vi "5 ch 12kHz only esonance scanner (FPGA) fixed pix clock.vi"() -> ()   [LabVIEW 2012]
uses:
  <vilib>/Platform/TimedLoop/XDataNode/timing_clust.ctl
  <vilib>/Platform/TimedLoop/XDataNode/nitl_modes.ctl
  <vilib>/Platform/TimedLoop/XDataNode/wakeup.ctl
  <vilib>/rvi/eio/common/nirviEmuTemplateMethod_errors.vi
  <vilib>/rvi/Emulation/niFpgaSctlEmulationRegisterWithScheduler.vi
  <vilib>/rvi/interface/RandomDataEmulation/nirviRandomDataFPGAFIFO.vi
  <vilib>/rvi/interface/RandomDataEmulation/niFpgaRandomDataHandleErrors.vi
  <vilib>/rvi/Emulation/niFpgaSctlEmulationScheduler.vi
  <vilib>/eio/EIONode/EIONode.xnode
  <vilib>/Platform/TimedLoop/XDataNode/XDataNode.xnode
  <vilib>/rvi/DataTransferAndStorage/Container/XNode/niFpgaContainer.xnode
  <vilib>/rvi/interface/RandomDataEmulation/nirviRandomDataFpgaReadWriteTemplate.vi
  <vilib>/Platform/TimedLoop/XDataNode/XDNodeRunTimeDep.lvlib
panel:
  in  "frequency (T:8kHz F:12kHz)":bool
  in  "lines at once":i16=4999
  in  "Start Delay (Ticks)":i16 caption="Start delay (Ticks)"
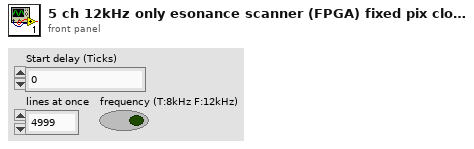
[diagram p1: front panel]
types:
  T1 = typedef "XDNodeRunTimeDep.lvlib/timing_clust.ctl" = cluster{"Expected End [f-1]":u64, "Actual End [f-1]":u64, "Finished Late? [f-1]":bool, "Expected End [i-1]":u64, "Actual End [i-1]":u64, "Finished Late? [i-1]":bool, "Expected Start [i]":u64, "Actual Start [i]":u64, "Expected Start [f]":u64, "Actual Start [f]":u64, "Source Name":string, "Structure Name":string, "Period":i64, "Deadline":i64, "Offset":i64, "Start":i64, "Priority":i32, "Timeout":i32, "Mode":T2, "Wakeup Reason":T3, "Error":errorcluster, "Source Type":string, "Secondary Source Type":string, "Global End Time":u64, "Global Start Time":u64, "Frame Duration":u64, "Iteration Duration":u64, "Assigned CPU":i32, "I/O Scan Engine Mode":u32}
  T2 = typedef "XDNodeRunTimeDep.lvlib/nitl_modes.ctl" = enum32{"No Change", "Process missed periods, maintain original phase", "Discard missed periods, maintain original phase", "Process missed periods, ignore original phase", "Discard missed periods, ignore original phase"}
  T3 = typedef "XDNodeRunTimeDep.lvlib/wakeup.ctl" = enum32{"Normal", "Aborted", "Asynchronous wakeup", "Timing source error", "Timed loop error", "Timeout"}
  T4 = cluster{"IO Module\\AI A0":i16, "IO Module\\AI A1":i16, "IO Module\\AI A3":i16, "IO Module\\AI A6":i16, "IO Module\\AI B8":i16}
  T5 = cluster{"IO Module\\AI A0":i32, "IO Module\\AI A1":i32, "IO Module\\AI A3":i32, "IO Module\\AI A6":i32, "IO Module\\AI B8":i32}
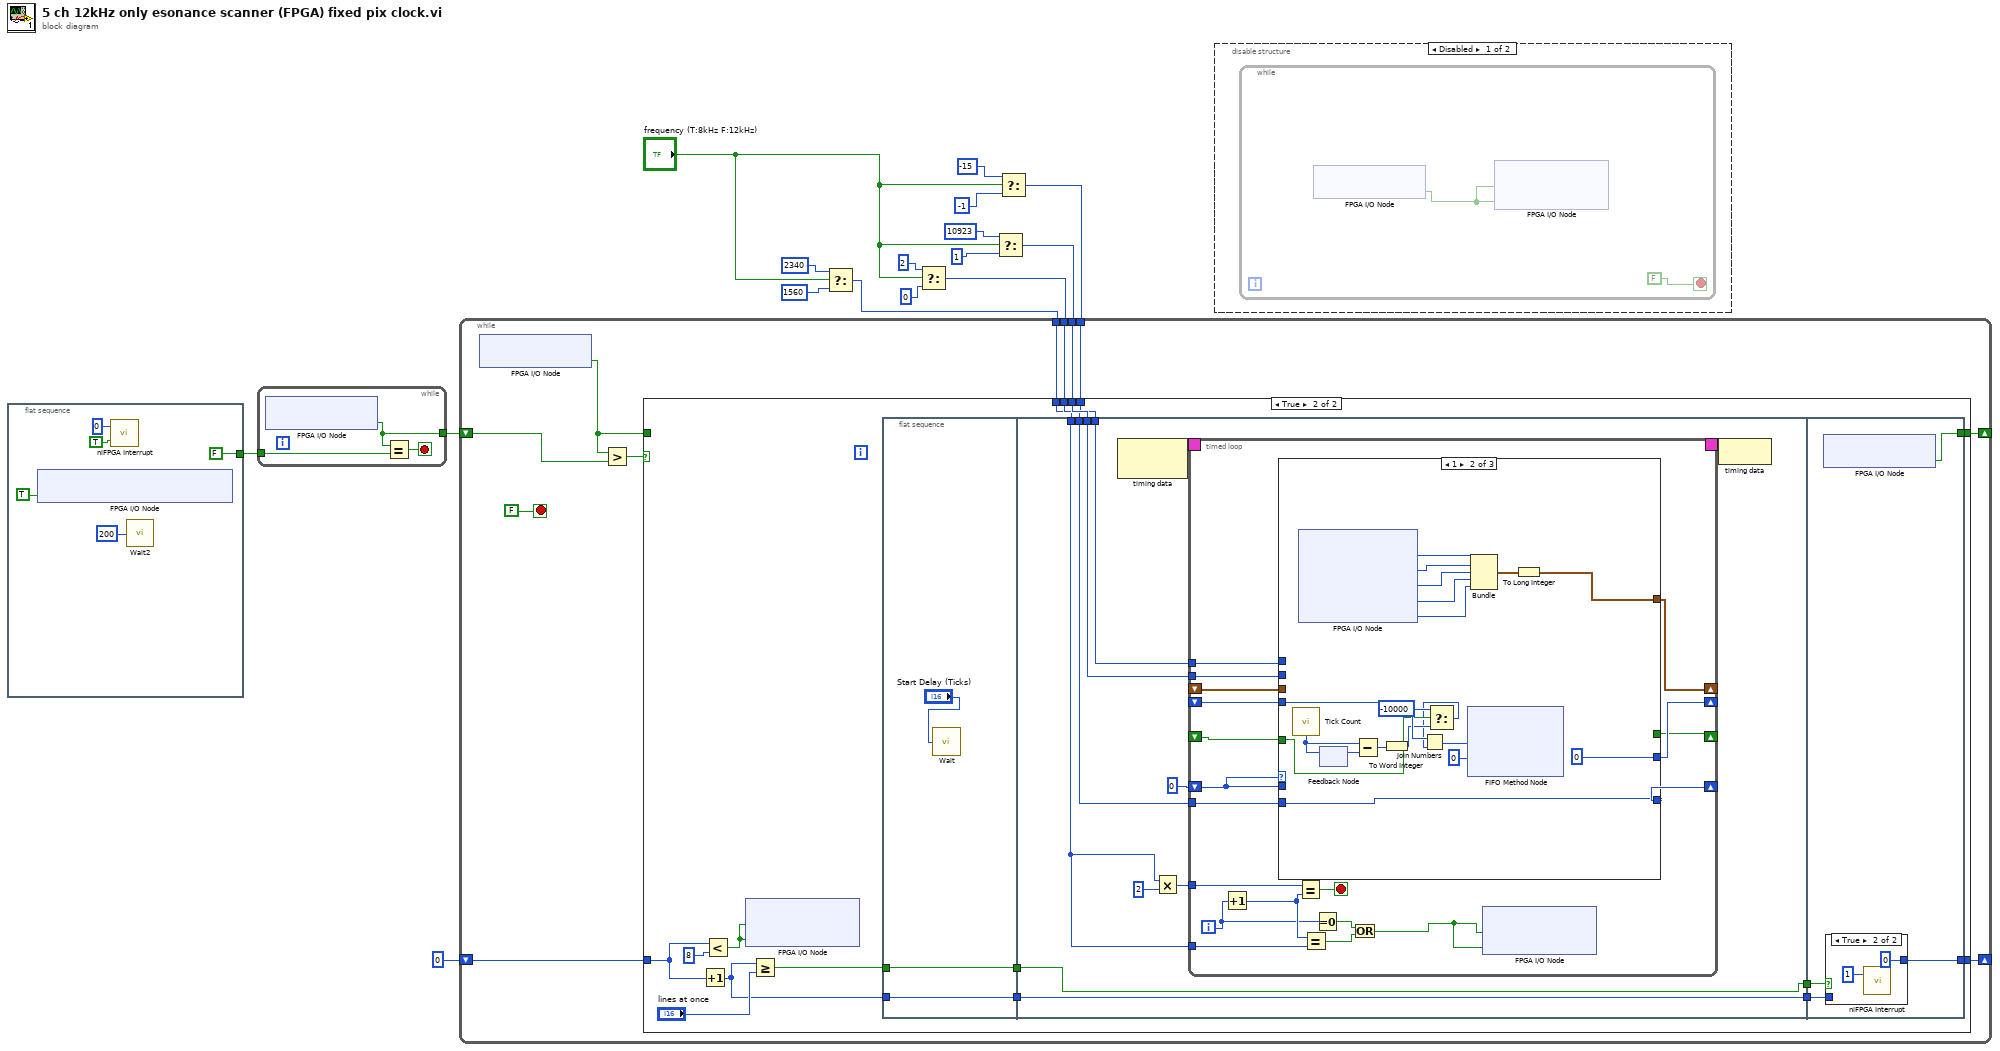
[diagram p0: block diagram]
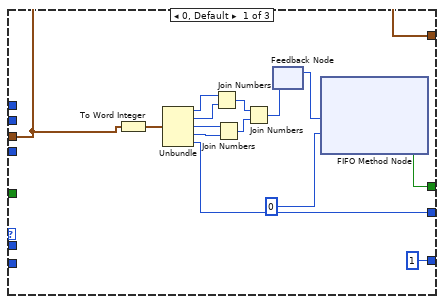
[diagram p4: hidden frame]
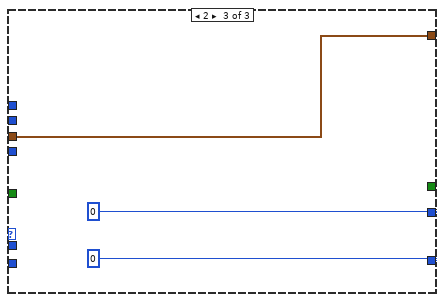
[diagram p5: hidden frame]
diagram:
  n1 = flat-sequence {
    tunnel: [FALSE ("IO Module\\DI 0")] -> w15
    frame #0 {
      n2 = xnode "FPGA I/O Node"("IO Module\\Digital Output Enable"=TRUE ("IO Module\\Digital Output Enable")) -> ()  [unwired: 1 in, 1 out]
      n3 = call <vilib>:"niFPGA Interrupt.vi"("Wait Until Cleared (F)"=TRUE, "IRQ Number (0)"=u8 0) -> ()  [unwired: 1 in]
      n4 = call "Wait2"("Count(mSec)"=u32 200) -> ()  [unwired: 1 out]
    }
  }
  n5 = while {
    tunnel: w15 -> [w24]
    tunnel: [w22] -> w14
    stop <- w23 stop-if-true
    n6 = xnode "FPGA I/O Node"() -> ("IO Module\\DI 0"=w22:bool)  [unwired: 1 in, 1 out]
    n7 = Equal?(x=w22, y=w24) -> (x = y?=w23:bool)
  }
  n8 = Select(t=i16 2340 ("samples per half period"), s="frequency (T:8kHz F:12kHz)", f=i16 1560 ("samples per half period")) -> (s? t:f=w1:i16)
  n9 = Select(t=i8 2 ("f"), s="frequency (T:8kHz F:12kHz)", f=i8 0 ("n")) -> (s? t:f=w5:i8)
  n10 = Select(t=i16 10923 ("n"), s="frequency (T:8kHz F:12kHz)", f=i16 1) -> (s? t:f=w7:i16)
  n11 = Select(t=i16 -15 ("n"), s="frequency (T:8kHz F:12kHz)", f=i16 -1 ("n")) -> (s? t:f=w6:i16)
  n12 = while {
    shift-right: [w34] -> _
    shift-left: w14 -> [w35]
    shift-right: [w32] -> _
    shift-left: i16 0 ("IRQ Number (0)") -> [w31]
    tunnel: w7 -> [w29]
    tunnel: w6 -> [w28]
    tunnel: w5 -> [w27]
    tunnel: w1 -> [w26]
    stop <- FALSE stop-if-true
    n13 = xnode "FPGA I/O Node"() -> ("IO Module\\DI 0"=w25:bool)  [unwired: 1 in, 1 out]
    n14 = Greater?(x=w25, y=w35) -> (0:w30:bool)
    n15 = case shown="True" w30 {
      tunnel: [w36 w50] -> w34
      tunnel: w31 -> [w37 w52]
      tunnel: [w37 w53] -> w32
      tunnel: w25 -> [w36 _]
      tunnel: w29 -> [_ w49]
      tunnel: w28 -> [_ w48]
      tunnel: w27 -> [_ w47]
      tunnel: w26 -> [_ w46]
      frame False {
      }
      frame True {
        n16 = Increment(x=w52) -> (x+1=w41:i16)
        n17 = Less?(x=w52, y=i16 8) -> (x < y?=w45:bool)
        n18 = xnode "FPGA I/O Node"("PXI_Trig2"=w45, "IO Module\\D0 2"=w45) -> ()  [unwired: 2 in, 2 out]
        n19 = Greater Or Equal?(x=w41, y="lines at once") -> (x >= y?=w38:bool)
        n20 = flat-sequence {
          tunnel: [w55] -> w42
          tunnel: w41 -> [w55]
          tunnel: [w54] -> w39
          tunnel: w38 -> [w54]
          tunnel: w49 -> [w62]
          tunnel: w48 -> [w61]
          tunnel: w47 -> [w60]
          tunnel: w46 -> [w59]
          tunnel: [w58] -> w43
          tunnel: w42 -> [w58]
          tunnel: [w57] -> w40
          tunnel: w39 -> [w57]
          tunnel: [w130] -> w53
          tunnel: [w129] -> w50
          tunnel: w43 -> [w128]
          tunnel: w40 -> [w127]
          frame #0 {
            n21 = call "Wait"("Count(Ticks)"="Start Delay (Ticks)") -> ()  [unwired: 1 out]
          }
          frame #1 {
            n22 = node-c288() -> (w65:T1)  [unwired: 1 in]
            n23 = Multiply(x=w59, y=i16 2) -> (x*y=w66:i16)
            n24 = timed-loop {
              tunnel: w66 -> [w85]
              timing: w65 -> [_]
              timing-out: [_] -> w64
              shift-right: [w84] -> _
              shift-left: i8 0 ("Timeout") -> [w74]
              tunnel: w59 -> [w80]
              shift-right: [w78] -> _
              shift-left: _ -> [w77]
              shift-right: [w76] -> _
              shift-left: _ -> [w75]
              tunnel: w62 -> [w73]
              tunnel: w61 -> [w72]
              tunnel: w60 -> [w71]
              shift-right: [w70] -> _
              shift-left: _ -> [w69]
              i -> [w79]
              stop <- w86 stop-if-true
              n25 = Increment(x=w79) -> (x+1=w81:i32)
              n26 = case shown="1" w74 {
                tunnel: w74 -> [_ _ _]
                tunnel: [i8 1 w102 i8 0] -> w84
                tunnel: [w87 w101 w120] -> w78
                tunnel: w77 -> [w87 _ w120]
                tunnel: [w92 i16 0 ("IO Module\\AI B8") i16 0 ("IO Module\\AI B8")] -> w76
                tunnel: w75 -> [_ w109 _]
                tunnel: w73 -> [_ _ _]
                tunnel: w72 -> [_ _ _]
                tunnel: w71 -> [_ w102 _]
                tunnel: [w90 _ _] -> w70
                tunnel: w69 -> [_ w105 _]
                frame 0, Default {
                  n27 = To Word Integer(number=w87) -> (16bit integer=w93:T4)
                  n28 = Unbundle(w93) -> ("IO Module\\AI A0"=w97:i16, "IO Module\\AI A1"=w96:i16, "IO Module\\AI A3"=w95:i16, "IO Module\\AI A6"=w94:i16, "IO Module\\AI B8"=w92:i16)
                  n29 = Join Numbers(hi=w97, lo=w96) -> ((hi.lo)=w98:u32)
                  n30 = Join Numbers(hi=w95, lo=w94) -> ((hi.lo)=w99:u32)
                  n31 = Join Numbers(hi=w98, lo=w99) -> ((hi.lo)=w91:u64)
                  n32 = feedback-in #1(w91) -> ()
                  n33 = feedback #1() -> (w89:u64)  [unwired: 1 in]
                  n34 = xnode ("FIFO Method Node")("Element"=w89, "Timeout"=0) -> ("Timed Out?"=w90:bool)  [unwired: 1 in, 1 out]
                }
                frame 1 {
                  n35 = call "Tick Count"() -> ("Tick Count(Ticks)"=w113:u32)
                  n36 = xnode "FPGA I/O Node"() -> ("IO Module\\AI A0"=w119:i16, "IO Module\\AI A1"=w118:i16, "IO Module\\AI A3"=w117:i16, "IO Module\\AI A6"=w116:i16, "IO Module\\AI B8"=w114:i16)  [unwired: 5 in, 5 out]
                  n37 = feedback #2() -> (w112:u32)  [unwired: 1 in]
                  n38 = feedback-in #2(w113) -> ()
                  n39 = Subtract(x=w113, y=w112) -> (x-y=w111:u32)
                  n40 = To Word Integer(number=w111) -> (16bit integer=w106:i16)
                  n41 = Select(t=i16 -10000, s=w105, f=w106) -> (s? t:f=w103:i16)
                  n42 = Join Numbers(hi=w109, lo=w103) -> ((hi.lo)=w107:u32)
                  n43 = xnode ("FIFO Method Node")("Element"=w107, "Timeout"=0) -> ()  [unwired: 1 in, 2 out]
                  n44 = Bundle("IO Module\\AI A0"=w119, "IO Module\\AI A1"=w118, "IO Module\\AI A3"=w117, "IO Module\\AI A6"=w116, "IO Module\\AI B8"=w114) -> (w115:T4)  [unwired: 1 in]
                  n45 = To Long Integer(number=w115) -> (32bit integer=w101:T5)
                }
                frame 2 {
                }
              }
              n46 = Equal?(x=w85, y=w81) -> (x = y?=w86:bool)
              n47 = Equal?(x=w81, y=w80) -> (x = y?=w82:bool)
              n48 = Equal To 0?(x=w79) -> (x = 0?=w83:bool)
              n49 = Or(x=w83, y=w82) -> (x .or. y?=w68:bool)
              n50 = xnode "FPGA I/O Node"("IO Module\\D0 1"=w68, "PXI_Trig1"=w68) -> ()  [unwired: 2 in, 2 out]
            }
            n51 = node-c288(w64) -> ()
          }
          frame #2 {
            n52 = xnode "FPGA I/O Node"() -> ("IO Module\\DI 0"=w129:bool)  [unwired: 1 in, 1 out]
            n53 = case shown="True" w127 {
              tunnel: w128 -> [w131 _]
              tunnel: [w131 u8 0] -> w130
              frame False {
              }
              frame True {
                n54 = call <vilib>:"niFPGA Interrupt.vi"("IRQ Number (0)"=u8 1) -> ()  [unwired: 2 in]
              }
            }
          }
        }
      }
    }
  }
  n55 = disable-structure shown="Disabled" {
    frame Disabled {
      n56 = while {
        stop <- FALSE stop-if-true
        n57 = xnode "FPGA I/O Node"() -> ("IO Module\\DI 0"=w135:bool)  [unwired: 1 in, 1 out]
        n58 = xnode "FPGA I/O Node"("IO Module\\D0 3"=w135, "PXI_Trig3"=w135) -> ()  [unwired: 2 in, 2 out]
      }
    }
    frame Enabled {
    }
  }
